vi "Replase ALR_ACKs.vi"(8 "error in (no error)":errorcluster, 9 "Ack":bool, 10 "Index":i32[](array[numeric]), 11 "ALR_ON_OFF":refnum<data-value>) -> (0 "error out":errorcluster, 3 "ALR_ON_OFF out":refnum<data-value>)   [LabVIEW 2019, in "Alarms.lvlib"]
uses:
  Alarms.lvlib
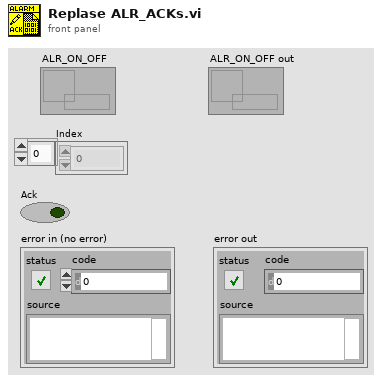
[diagram p1: front panel]
types:
  T1 = cluster{"ALR_ON":bool[], "ALR_OFF":bool[], "ALR_reset":bool[], "ALR_check":bool[], "ALR_block":bool[], "ALR_Ack":bool[]}
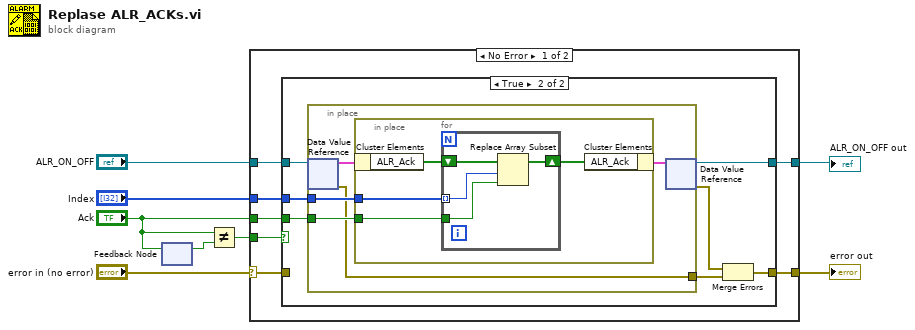
[diagram p0: block diagram]
diagram:
  n1 = feedback #1() -> (w3:bool)  [unwired: 1 in]
  n2 = feedback-in #1("Ack") -> ()
  n3 = Not Equal?(x="Ack", y=w3) -> (x != y?=w1:bool)
  n4 = case shown="No Error" "error in (no error)" {
    selector: "error in (no error)" -> [w11 w39]
    tunnel: "Index" -> [w15 _]
    tunnel: [w12 w39] -> w7
    tunnel: "ALR_ON_OFF" -> [w14 w38]
    tunnel: [w9 w38] -> w5
    tunnel: "Ack" -> [w13 _]
    tunnel: w1 -> [w10 _]
    frame No Error {
      n5 = case shown="True" w10 {
        tunnel: w15 -> [_ w24]
        tunnel: w14 -> [w16 w23]
        tunnel: w13 -> [_ w22]
        tunnel: [w17 w19] -> w12
        tunnel: w11 -> [w17 _]
        tunnel: [w16 w18] -> w9
        frame False {
        }
        frame True {
          n6 = in-place {
            in-place-border: w24 -> [w28]
            in-place-border: w22 -> [w27]
            in-place-border: [w25] -> w20
            n7 = in-place-dvr #2(w23) -> (w29:T1, w25:errorcluster)
            n8 = in-place {
              in-place-border: w28 -> [w32]
              in-place-border: w27 -> [w31]
              n9 = in-place-cluster #3(w29) -> ("ALR_Ack"=w33:bool[])
              n10 = for {
                tunnel: w32 -> [w36] mode=indexing
                tunnel: w31 -> [w35]
                shift-right: [w34] -> w30
                shift-left: w33 -> [w37]
                n11 = Replace Array Subset(array=w37, new element=w35, index=w36) -> (w34:bool[])
              }
              n12 = in-place-cluster #3("ALR_Ack"=w30) -> (w26:T1)
            }
            n13 = in-place-dvr #2(w26) -> (w18:refnum<data-value>, w21:errorcluster)
          }
          n14 = Merge Errors(w21, w20) -> (w19:errorcluster)
        }
      }
    }
    frame Error {
    }
  }
  "error out" <- w7
  "ALR_ON_OFF out" <- w5
